vi "find and open select worksheet.vi"(7 "Worksheet Names":string[](array[string]), 8 "error in (no error)":errorcluster, 9 "milliseconds to wait":u32=100, 10 "Worksheet Name in":string, 11 "NI_report in":refnum<class "NI_report.lvclass">) -> (0 "error out":errorcluster, 2 "Select Worksheet Index":i32, 3 "NI_report out":refnum<class "NI_report.lvclass">)   [LabVIEW 2016]
uses:
  <vilib>/Utility/NIReport.llb/NI_report.lvclass
  <vilib>/Utility/NIReport.llb/Excel/NI_Excel.lvclass
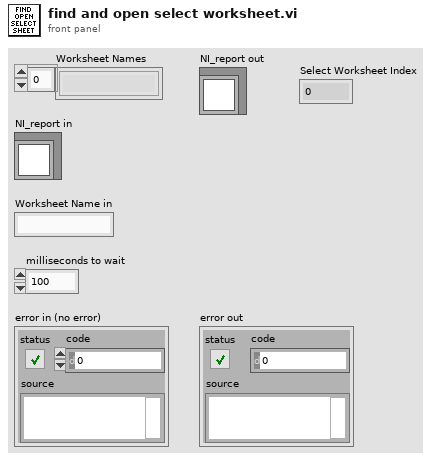
[diagram p1: front panel]
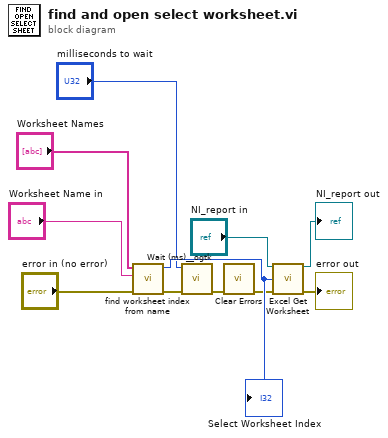
[diagram p0: block diagram]
diagram:
  n1 = call "find worksheet index from name.vi"("error in (no error)"="error in (no error)", "Worksheet Name in"="Worksheet Name in", "Worksheet Names"="Worksheet Names") -> ("error out"=w10:errorcluster, "Select Worksheet Index"=w8:i32)  [unwired: 7 in]
  "Select Worksheet Index" <- w8
  n2 = call "Wait (ms)__ogtk.vi"("error in (no error)"=w10, "milliseconds to wait"="milliseconds to wait") -> ("error out"=w1:errorcluster)  [unwired: 8 in, 1 out]
  n3 = call <vilib>:"Clear Errors.vi"("error in (no error)"=w1) -> ("error out"=w3:errorcluster)  [unwired: 5 in, 1 out]
  n4 = call <vilib>:"Excel Get Worksheet.vi"("report in"="NI_report in", "worksheet index (0)"=w8, "error in (no error)"=w3) -> ("report out"=→"NI_report out":refnum<class "NI_report.lvclass">, "error out"=→"error out":errorcluster)  [unwired: 11 in]
